vi "Main.vi"(8 "error in":errorcluster, 9 ">>ErrorQ":refnum<queue>, 11 ">>EventHandlers":refnum<user-event>) -> (0 "error out":errorcluster)   [LabVIEW 2020, in "UserConsole.lvlib"]
doc: "This is a template for creating new VIs for the owning library"
uses:
  UserConsole.lvlib
  Error Handler/Controls/Error QMsg.ctl
  Support/Controls/Project Modules.ctl
  Support/Controls/Project Event Msg.ctl
  Support/Controls/Project Events.ctl
  Controls/Operational Loop Data.ctl
  Controls/Module QMsg.ctl
  Support/Support.lvlib
  Controls/Module Event Msg.ctl
  Error Handler/ErrorHandler.lvlib
panel:
  in  "Elevator Call":T1
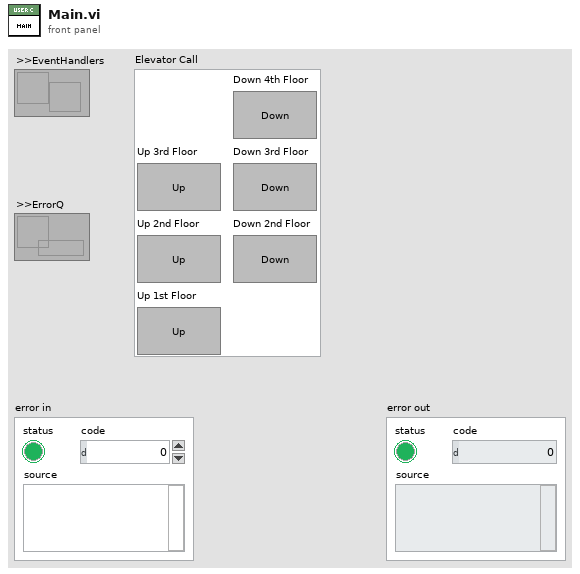
[diagram p1: front panel]
types:
  T1 = cluster{"Down 4th Floor":bool, "Down 3rd Floor":bool, "Down 2nd Floor":bool, "Up 1st Floor":bool, "Up 3rd Floor":bool, "Up 2nd Floor":bool}
  T2 = typedef "Support.lvlib/Project Events.ctl" = enum16{"Stop", "Initialize", "Elevator Call"}
  T3 = typedef "UserConsole.lvlib/Module QMsg.ctl" = cluster{"Command":string, "Data":variant}
  T4 = typedef "UserConsole.lvlib/Operational Loop Data.ctl" = cluster{"Dummy":dbl}
  T5 = typedef "UserConsole.lvlib/Module Messaging Structures.ctl" = cluster{">>EventHandlers":refnum<user-event>, ">>ErrorQ":refnum<queue>}
  T6 = typedef "UserConsole.lvlib/Module Event Msg.ctl" = cluster{"Command":string, "Data":variant}
  T7 = typedef "Support.lvlib/Project Event Msg.ctl" = cluster{"Command":string, "Data":variant, "Events":T2}
  T8 = cluster{"Direction is Up?":bool, "Current Floor":i32}
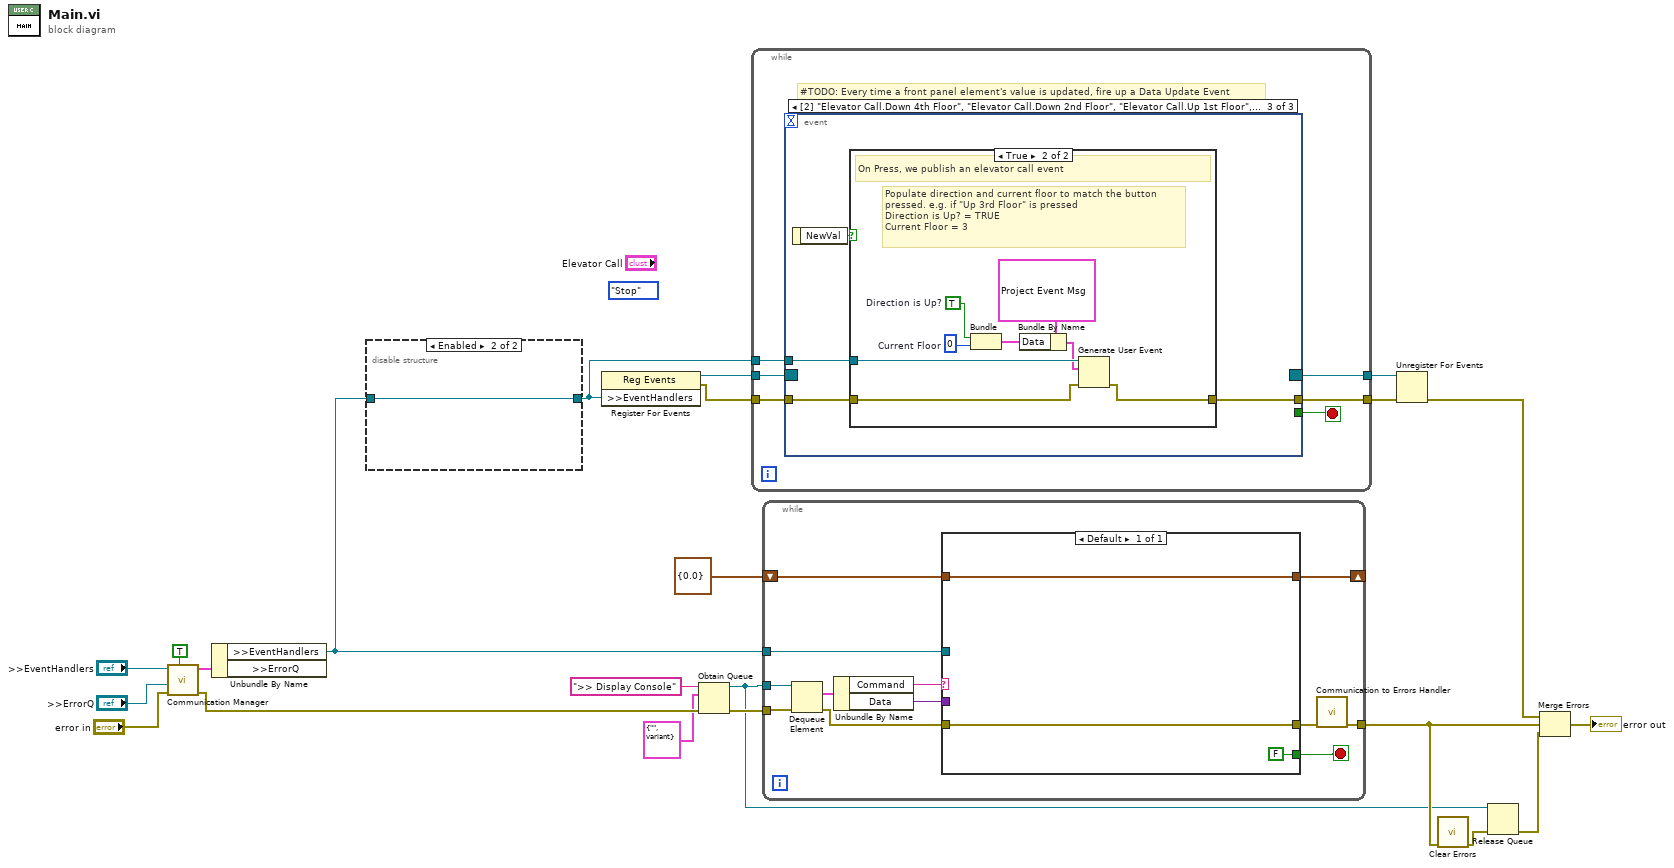
[diagram p0: block diagram]
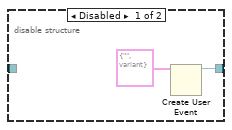
[diagram p2: hidden frame]
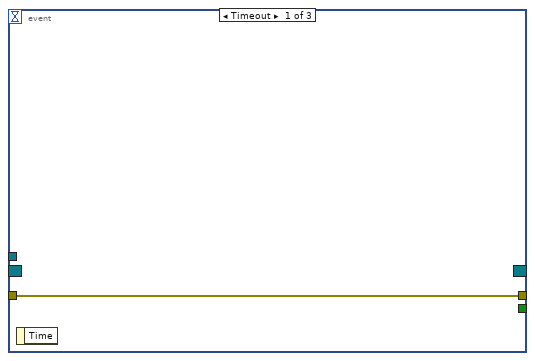
[diagram p3: hidden frame]
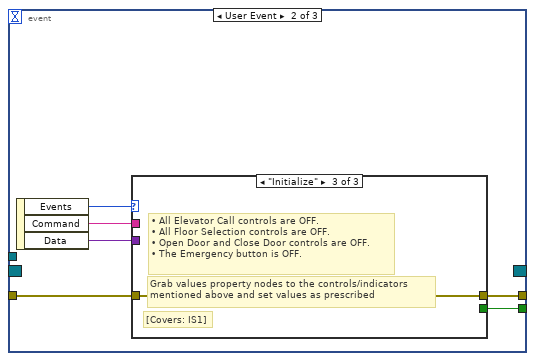
[diagram p4: hidden frame]
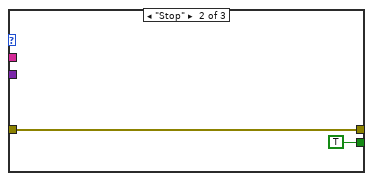
[diagram p6: hidden frame]
diagram:
  (unwired) Project_Events."Stop" ("Events")
  n1 = call "Communication Manager.vi"("Load?"=TRUE, "error in"="error in", ">>ErrorQ"=">>ErrorQ", ">>EventHandlers"=">>EventHandlers") -> ("error out"=w8:errorcluster, "Messaging Structures"=w18:T5)  [unwired: 6 in]
  n2 = Unbundle By Name(w18) -> (">>EventHandlers"=w11:refnum<user-event>)  [unwired: 1 out]
  n3 = disable-structure shown="Enabled" {
    disable-tunnel: w11 -> [_ w25]
    disable-tunnel: [w23 w25] -> w10
    frame Disabled {
      n4 = Create User Event(user event datatype=T6 {"Command"="", "Data"=variant} ("QMessage")) -> (user event=w23:refnum<user-event>)  [unwired: 1 in, 1 out]
    }
    frame Enabled {
    }
  }
  n5 = register-events(w10) -> (reference out=w17:refnum<event-registration>, error out=w15:errorcluster)  [unwired: 2 in]
  n6 = Obtain Queue(name (unnamed)=">> Display Console", element data type=T3 {"Command"="", "Data"=variant} ("QMessage"), error in (no error)=w8) -> (queue out=w2:refnum<queue>, error out=w9:errorcluster)  [unwired: 2 in, 1 out]
  n7 = while {
    tunnel: w10 -> [w31]
    tunnel: w17 -> [w30]
    tunnel: [w29] -> w16
    tunnel: w15 -> [w28]
    tunnel: [w27] -> w14
    stop <- w26 stop-if-true
    # "#TODO: Every time a front panel element's value is updated, fire up a Data Update Event"
    n8 = event shown="[2] \"Elevator Call.Down 4th Floor\", \"Elevator Call.Down 2nd Floor\", \"Elevator Call.Up 1st Floor\", \"Elevator Call.Up 3rd Floor\", \"Elevator Call.Up 2nd Floor\": Value Change" {
      selector: w30 -> [_ _ _]
      dyn-events: [_ _ _] -> w29
      timeout: _ -> [_ _ _]
      tunnel: w31 -> [_ _ w43]
      tunnel: w28 -> [w32 w38 w45]
      tunnel: [w32 w37 w44] -> w27
      tunnel: [_ w35 _] -> w26
      event Timeout {
        n9 = event-data() -> ()  [unwired: 1 in, 1 out]
      }
      event User Event {
        n10 = event-data() -> ("Events"=w36:T2, "Command"=w34:string, "Data"=w33:variant)  [unwired: 1 in]
        n11 = case shown="\"Initialize\"" w36 {
          tunnel: w38 -> [w39 w41 w42]
          tunnel: [w39 w41 w42] -> w37
          tunnel: [_ TRUE _] -> w35
          tunnel: w34 -> [_ _ _]
          tunnel: w33 -> [_ _ _]
          frame Default {
          }
          frame "Stop" {
          }
          frame "Initialize" {
            # "[Covers: IS1]"
            # "Grab values property nodes to the controls/indicators \nmentioned above and set values as prescribed"
            # "• All Elevator Call controls are OFF.\n• All Floor Selection controls are OFF.\n• Open Door and Close Door controls are OFF.\n• The Emergency button is OFF."
          }
        }
      }
      event "Elevator Call.Down 4th Floor", "Elevator Call.Down 2nd Floor", "Elevator Call.Up 1st Floor", "Elevator Call.Up 3rd Floor", "Elevator Call.Up 2nd Floor": Value Change {
        n12 = event-data() -> ("NewVal"=w46:bool)  [unwired: 1 in]
        n13 = case shown="True" w46 {
          tunnel: w45 -> [w47 w54]
          tunnel: [w47 w53] -> w44
          tunnel: w43 -> [_ w55]
          frame False {
          }
          frame True {
            w48 = 0  # Current Floor
            w49 = TRUE  # Direction is Up?
            # "Populate direction and current floor to match the button\npressed. e.g. if \"Up 3rd Floor\" is pressed \nDirection is Up? = TRUE\nCurrent Floor = 3"
            # "On Press, we publish an elevator call event"
            n14 = Bundle("Direction is Up?"=w49, "Current Floor"=w48) -> (w50:T8)  [unwired: 1 in]
            n15 = Bundle By Name(cluster=T7 {"Command"="", "Data"=variant, "Events"=enum."Elevator Call"} ("event data"), "Data"=w50) -> (w51:T7)
            n16 = Generate User Event(user event=w55, event data cluster=w51, error in=w54) -> (error out=w53:errorcluster)  [unwired: 1 in, 1 out]
          }
        }
      }
    }
  }
  n17 = while {
    tunnel: w2 -> [w67]
    tunnel: w11 -> [w60]
    tunnel: w9 -> [w66]
    tunnel: [w58] -> w3
    shift-right: [w56] -> _
    shift-left: T4 {"Dummy"=0.0} ("Operation Loop Data") -> [w57]
    stop <- w62 stop-if-true
    n18 = Dequeue Element(queue=w67, error in (no error)=w66) -> (element=w65:T3, error out=w61:errorcluster)  [unwired: 1 in, 2 out]
    n19 = Unbundle By Name(w65) -> ("Command"=w64:string, "Data"=w63:variant)
    n20 = case shown="Default" w64 {
      tunnel: w63 -> [_]
      tunnel: [FALSE] -> w62
      tunnel: w61 -> [w70]
      tunnel: [w70] -> w59
      tunnel: w60 -> [_]
      tunnel: w57 -> [w69]
      tunnel: [w69] -> w56
      frame Default {
      }
    }
    n21 = call "Communication to Errors Handler.vi"("error in"=w59) -> ("error out"=w58:errorcluster)  [unwired: 10 in]
  }
  n22 = Unregister For Events(event registration refnum=w16, error in=w14) -> (error out=w13:errorcluster)
  n23 = call <vilib>:"Clear Errors.vi"("error in (no error)"=w3) -> ("error out"=w4:errorcluster)  [unwired: 5 in, 1 out]
  n24 = Release Queue(queue=w2, error in (no error)=w4) -> (error out=w1:errorcluster)  [unwired: 1 in, 2 out]
  n25 = Merge Errors(w13, w3, w1) -> (→"error out":errorcluster)
